vi "_RT_CtrlLoop_TurboPump.vi"(6 "ExpVar in":refnum<class "ExpVar.lvclass">, 8 "error in (no error)":errorcluster, 10 "safty":refnum<data-value>) -> ()   [LabVIEW 2018]
uses:
  PublicSubVI/NewExpVar/ExpVar.lvclass
  Ctl/Function_of_TC110.ctl
  PublicSubVI/Ctl/_ctl_RT_TurboSettings.ctl
  PublicSubVI/Ctl/_ctl_RT_SysLog.ctl
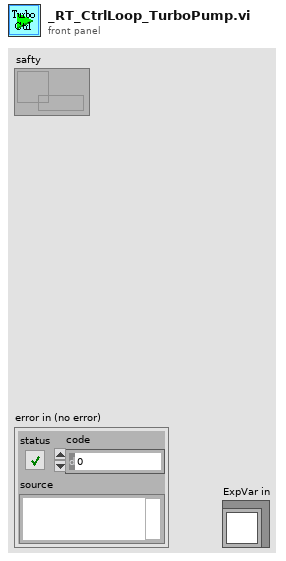
[diagram p1: front panel]
types:
  T1 = typedef "Function_of_TC110.ctl" = enum16{"Initialisation", "Read status", "Write command", "Read command"}
  T2 = cluster{"Speed":dbl, "Power":dbl, "rot. speed":dbl}
  T3 = enum16{"via string label", "Laser", "Pressure", "TMP", "Script", "Signal Remarks", "ExtAO", "ExtDO", "ExtDI", "D999"}
  T4 = typedef "_ctl_RT_SysLog.ctl" = enum16{"None", "Initialize", "StartupRT", "StartupFPGA", "StartupAllocator", "GetMass", "SetWfmCode", "SetLaserCtrl", "SetTurboCtrl", "SetD999Ctrl", "Reconnecting...", "Interrupt", "StopRT"}
  T5 = typedef "_ctl_RT_TurboSettings.ctl" = cluster{"Preset rot. speed \nat standby mode(%)":dbl, "Speed set value in rot. speed \nsetting operations (%)":dbl, "Max. power (%)":dbl, "Gas mode: ":enum16{"heavy", "light", "helium"}, "Operations mode: ":bool, "Motor turbopump: ":bool, "Pumping station: ":bool, "Standby: ":bool, "Timestamp":timestamp}
  T6 = cluster{"Motor voltage":string, "Actual power":string, "Target speed":string, "Actual speed":string, "Temp. of electronics":string, "Temp. of pump bottom":string}
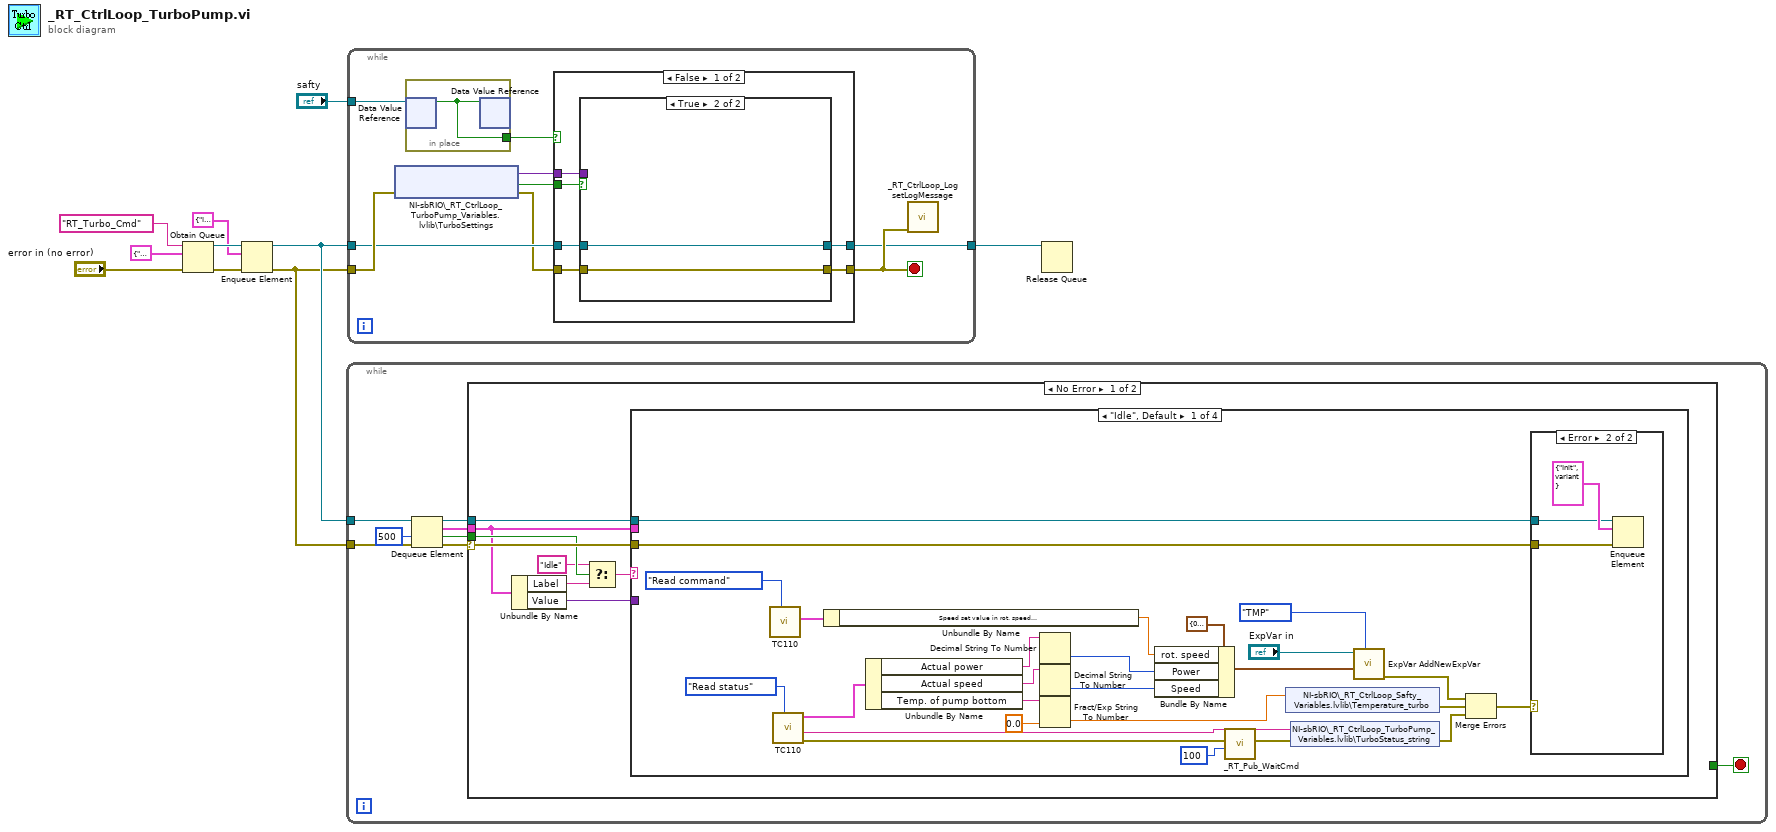
[diagram p0: block diagram]
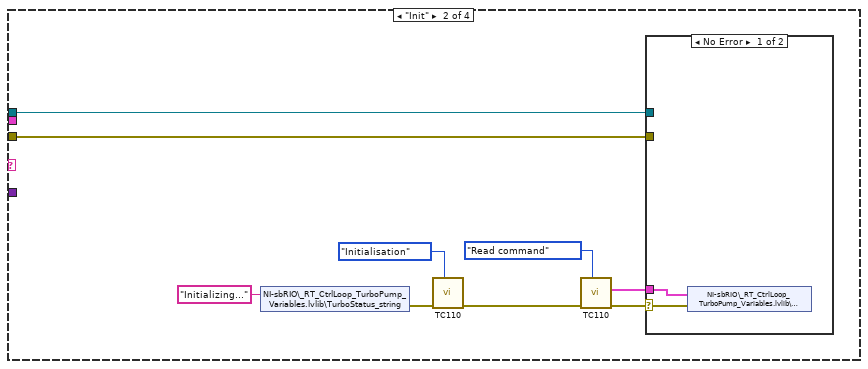
[diagram p3: hidden frame]
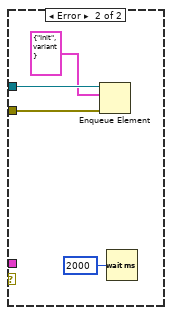
[diagram p4: hidden frame]
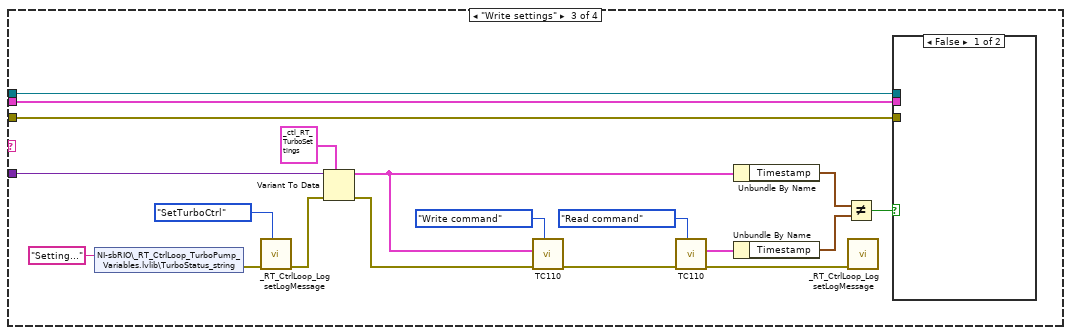
[diagram p5: hidden frame]
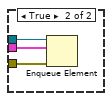
[diagram p6: hidden frame]
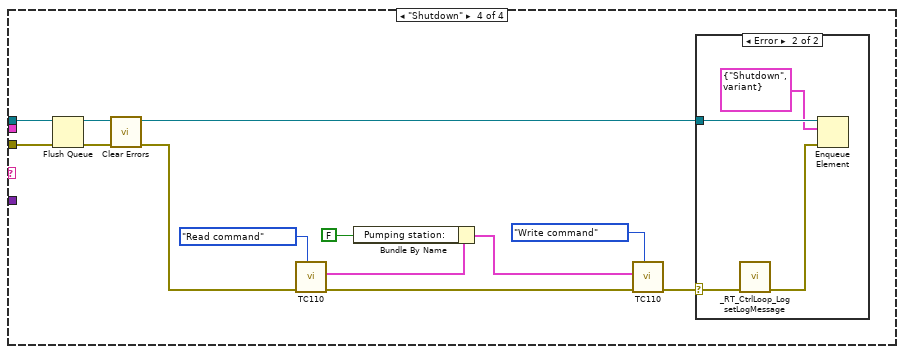
[diagram p7: hidden frame]
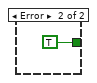
[diagram p9: hidden frame]
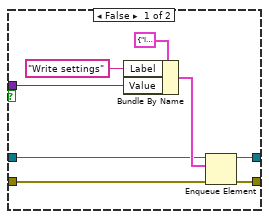
[diagram p10: hidden frame]
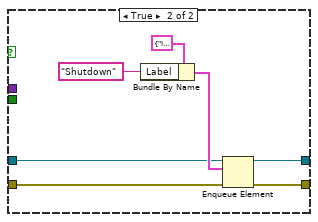
[diagram p11: hidden frame]
diagram:
  n1 = Obtain Queue(name (unnamed)="RT_Turbo_Cmd", element data type=cluster{"Label":string, "Value":variant} {"Label"="", "Value"=variant}, error in (no error)="error in (no error)") -> (queue out=w7:refnum<queue>, error out=w6:errorcluster)  [unwired: 2 in, 1 out]
  n2 = Enqueue Element(queue=w7, element=cluster{"Label":string, "Value":variant} {"Label"="Init", "Value"=variant}, error in (no error)=w6) -> (queue out=w3:refnum<queue>, error out=w2:errorcluster)  [unwired: 1 in, 1 out]
  n3 = while {
    tunnel: w3 -> [w18]
    tunnel: w2 -> [w17]
    stop <- w11 stop-if-true
    n4 = Dequeue Element(queue=w18, timeout in ms (-1)=500, error in (no error)=w17) -> (queue out=w15:refnum<queue>, element=w16:cluster{"Label":string, "Value":variant}, timed out?=w12:bool, error out=w14:errorcluster)
    n5 = case shown="No Error" w14 {
      selector: w14 -> [w24 _]
      tunnel: w16 -> [w19 _]
      tunnel: w15 -> [w25 _]
      tunnel: w12 -> [w23 _]
      tunnel: [_ TRUE] -> w11
      frame No Error {
        n6 = Unbundle By Name(w19) -> ("Label"=w22:string, "Value"=w26:variant)
        n7 = Select(t="Idle", s=w23, f=w22) -> (s? t:f=w20:string)
        n8 = case shown="\"Idle\", Default" w20 {
          tunnel: w26 -> [_ _ w74 _]
          tunnel: w24 -> [w27 w63 w76 w97]
          tunnel: w25 -> [w28 w64 w78 w98]
          tunnel: w19 -> [_ _ w77 _]
          frame "Idle", Default {
            n9 = call "TC110.vi"("Function"=Function_of_TC110."Read command") -> ("Settings out"=w36:T5)  [unwired: 7 in, 3 out]
            n10 = call "TC110.vi"("Function"=Function_of_TC110."Read status") -> ("Error out"=w46:errorcluster, "Status_string"=w52:string, "output cluster"=w51:T6)  [unwired: 7 in, 1 out]
            n11 = Unbundle By Name(w36) -> ("Speed set value in rot. speed \nsetting operations (%)"=w37:dbl)
            n12 = Unbundle By Name(w51) -> ("Actual power"=w50:string, "Actual speed"=w49:string, "Temp. of pump bottom"=w48:string)
            n13 = Decimal String To Number(string=w50) -> (number=w39:i32)  [unwired: 2 in, 1 out]
            n14 = Decimal String To Number(string=w49) -> (number=w38:i32)  [unwired: 2 in, 1 out]
            n15 = Fract/Exp String To Number(string=w48, default (0 dbl)=sgl 0.0 ("default (0 DBL)")) -> (number=w47:sgl)  [unwired: 2 in, 1 out]
            n16 = Bundle By Name(cluster=T2 {"Speed"=0.0, "Power"=0.0, "rot. speed"=0.0} ("TMP"), "rot. speed"=w37, "Power"=w39, "Speed"=w38) -> (w41:T2)
            n17 = call "_RT_Pub_WaitCmd.vi"("milliseconds to wait"=u32 100, "error in (no error)"=w46) -> ("error out"=w45:errorcluster)  [unwired: 9 in]
            n18 = shared-variable "NI-sbRIO\\_RT_CtrlLoop_Safty_Variables.lvlib\\Temperature_turbo"(w47) -> (error out=w44:errorcluster)  [unwired: 1 in]
            n19 = shared-variable "NI-sbRIO\\_RT_CtrlLoop_TurboPump_Variables.lvlib\\TurboStatus_string"(w52, error in=w45) -> (error out=w43:errorcluster)
            n20 = call-dynamic "ExpVar AddNewExpVar.vi"("VarType"=T3."TMP", "Var"=w41, "ExpVar in"="ExpVar in") -> ("error out"=w42:errorcluster)  [unwired: 7 in, 1 out]
            n21 = Merge Errors(w42, w44, w43) -> (w29:errorcluster)
            n22 = case shown="Error" w29 {
              tunnel: w28 -> [_ w54]
              tunnel: w27 -> [_ w53]
              frame No Error {
              }
              frame Error {
                n23 = Enqueue Element(queue=w54, element=cluster{"Label":string, "Value":variant} {"Label"="Init", "Value"=variant}, error in (no error)=w53) -> ()  [unwired: 1 in, 3 out]
              }
            }
          }
          frame "Init" {
            n24 = shared-variable "NI-sbRIO\\_RT_CtrlLoop_TurboPump_Variables.lvlib\\TurboStatus_string"("Initializing..." ("TurboStatus_string")) -> (error out=w56:errorcluster)  [unwired: 1 in]
            n25 = call "TC110.vi"("Function"=Function_of_TC110."Initialisation", "Error in"=w56) -> ("Error out"=w62:errorcluster)  [unwired: 6 in, 3 out]
            n26 = call "TC110.vi"("Function"=Function_of_TC110."Read command", "Error in"=w62) -> ("Error out"=w59:errorcluster, "Settings out"=w58:T5)  [unwired: 6 in, 2 out]
            n27 = case shown="No Error" w59 {
              selector: w59 -> [w66 _]
              tunnel: w64 -> [_ w70]
              tunnel: w63 -> [_ w69]
              tunnel: w58 -> [w65 _]
              frame No Error {
                n28 = shared-variable "NI-sbRIO\\_RT_CtrlLoop_TurboPump_Variables.lvlib\\TurboSettings"(w65, error in=w66) -> ()  [unwired: 1 out]
              }
              frame Error {
                n29 = Enqueue Element(queue=w70, element=cluster{"Label":string, "Value":variant} {"Label"="Init", "Value"=variant}, error in (no error)=w69) -> ()  [unwired: 1 in, 3 out]
                n30 = Wait (ms)(milliseconds to wait=u32 2000) -> ()  [unwired: 1 out]
              }
            }
          }
          frame "Write settings" {
            n31 = shared-variable "NI-sbRIO\\_RT_CtrlLoop_TurboPump_Variables.lvlib\\TurboStatus_string"("Setting..." ("TurboStatus_string")) -> (error out=w84:errorcluster)  [unwired: 1 in]
            n32 = call "_RT_CtrlLoop_Log setLogMessage.vi"("system type"=_ctl_RT_SysLog."SetTurboCtrl", "error in"=w84) -> ("error out"=w75:errorcluster)  [unwired: 8 in, 1 out]
            n33 = Variant To Data(error in=w75, type=T5 {"Preset rot. speed \nat standby mode(%)"=0.0, "Speed set value in rot. speed \nsetting operations (%)"=0.0, "Max. power (%)"=0.0, "Gas mode: "=enum."heavy", "Operations mode: "=FALSE, "Motor turbopump: "=FALSE, "Pumping station: "=FALSE, "Standby: "=FALSE, "Timestamp"=timestamp(0 s since 1904-01-01)} ("TurboSettings"), Variant=w74) -> (data=w82:T5, error out=w89:errorcluster)
            n34 = call "TC110.vi"("Function"=Function_of_TC110."Write command", "Error in"=w89, "Settings in"=w82) -> ("Error out"=w72:errorcluster)  [unwired: 5 in, 3 out]
            n35 = call "TC110.vi"("Function"=Function_of_TC110."Read command", "Error in"=w72) -> ("Error out"=w71:errorcluster, "Settings out"=w81:T5)  [unwired: 6 in, 2 out]
            n36 = Unbundle By Name(w82) -> ("Timestamp"=w80:timestamp)
            n37 = Unbundle By Name(w81) -> ("Timestamp"=w73:timestamp)
            n38 = Not Equal?(x=w80, y=w73) -> (x != y?=w79:bool)
            n39 = call "_RT_CtrlLoop_Log setLogMessage.vi"("error in"=w71) -> ()  [unwired: 9 in, 2 out]
            n40 = case shown="False" w79 {
              tunnel: w78 -> [_ w92]
              tunnel: w77 -> [_ w91]
              tunnel: w76 -> [_ w90]
              frame False {
              }
              frame True {
                n41 = Enqueue Element(queue=w92, element=w91, error in (no error)=w90) -> ()  [unwired: 1 in, 3 out]
              }
            }
          }
          frame "Shutdown" {
            n42 = Flush Queue(queue=w98, error in (no error)=w97) -> (queue out=w94:refnum<queue>, error out=w96:errorcluster)  [unwired: 1 out]
            n43 = call <vilib>:"Clear Errors.vi"("error in (no error)"=w96) -> ("error out"=w93:errorcluster)  [unwired: 5 in, 1 out]
            n44 = call "TC110.vi"("Function"=Function_of_TC110."Read command", "Error in"=w93) -> ("Error out"=w104:errorcluster, "Settings out"=w103:T5)  [unwired: 6 in, 2 out]
            n45 = Bundle By Name(cluster=w103, "Pumping station:"=FALSE) -> (w102:T5)
            n46 = call "TC110.vi"("Function"=Function_of_TC110."Write command", "Error in"=w104, "Settings in"=w102) -> ("Error out"=w95:errorcluster)  [unwired: 5 in, 3 out]
            n47 = case shown="Error" w95 {
              selector: w95 -> [_ w106]
              tunnel: w94 -> [_ w108]
              frame No Error {
              }
              frame Error {
                n48 = call "_RT_CtrlLoop_Log setLogMessage.vi"("error in"=w106) -> ("error out"=w105:errorcluster)  [unwired: 9 in, 1 out]
                n49 = Enqueue Element(queue=w108, element=cluster{"Label":string, "Value":variant} {"Label"="Shutdown", "Value"=variant}, error in (no error)=w105) -> ()  [unwired: 1 in, 3 out]
              }
            }
          }
        }
      }
      frame Error {
      }
    }
  }
  n50 = while {
    tunnel: "safty" -> [w118]
    tunnel: w2 -> [w114]
    tunnel: w3 -> [w113]
    tunnel: [w110] -> w1
    stop <- w111 stop-if-true
    n51 = shared-variable "NI-sbRIO\\_RT_CtrlLoop_TurboPump_Variables.lvlib\\TurboSettings"(error in=w114) -> (w115:variant, error out=w112:errorcluster, w116:bool)  [unwired: 1 in]
    n52 = in-place {
      in-place-border: [w142] -> w117
      n53 = in-place-dvr #1(w118) -> (w142:bool)  [unwired: 1 out]
      n54 = in-place-dvr #1(w142) -> ()  [unwired: 2 out]
    }
    n55 = case shown="False" w117 {
      tunnel: w116 -> [w124 _]
      tunnel: w115 -> [w123 _]
      tunnel: w113 -> [w122 w138]
      tunnel: w112 -> [w121 w137]
      tunnel: [w119 w135] -> w111
      tunnel: [w120 w136] -> w110
      frame False {
        n56 = case shown="True" w124 {
          tunnel: w123 -> [w130 _]
          tunnel: w122 -> [w128 w134]
          tunnel: w121 -> [w127 w133]
          tunnel: [w126 w134] -> w120
          tunnel: [w125 w133] -> w119
          frame False {
            n57 = Bundle By Name(cluster=cluster{"Label":string, "Value":variant} {"Label"="Init", "Value"=variant} ("element"), "Label"="Write settings", "Value"=w130) -> (w129:cluster{"Label":string, "Value":variant})
            n58 = Enqueue Element(queue=w128, element=w129, error in (no error)=w127) -> (queue out=w126:refnum<queue>, error out=w125:errorcluster)  [unwired: 1 in, 1 out]
          }
          frame True {
          }
        }
      }
      frame True {
        n59 = Bundle By Name(cluster=cluster{"Label":string, "Value":variant} {"Label"="Init", "Value"=variant} ("element"), "Label"="Shutdown") -> (w139:cluster{"Label":string, "Value":variant})
        n60 = Enqueue Element(queue=w138, element=w139, error in (no error)=w137) -> (queue out=w136:refnum<queue>, error out=w135:errorcluster)  [unwired: 1 in, 1 out]
      }
    }
    n61 = call "_RT_CtrlLoop_Log setLogMessage.vi"("error in"=w111) -> ()  [unwired: 9 in, 2 out]
  }
  n62 = Release Queue(queue=w1) -> ()  [unwired: 2 in, 3 out]
